vi "Test-Elevator Motors-Percent.vi"() -> ()   [LabVIEW 2014, in "Dev Elevator.lvlib"]
uses:
  Dev Robot/Dev Elevator/Dev Elevator.lvlib
  Robot Actor Framework/Trace/Trace Controller Class/Config.ctl
  Comp Motors with Encoders/Comp Motors with Encoders Class/Motor Controller Config.ctl
  Robot/Motor with Encoders/Motors with Encoders Class/Motors with Encoders Config.ctl
  Comp Motors with Encoders/Comp Motors with Encoders Class/Encoder Config.ctl
  Comp Trace Controller/Comp Trace Controller Class/Comp Trace Controller.lvclass
  Comp Pressure/Comp Pressure Class/Comp Pressure.lvclass
  <vilib>/Rock Robotics/WPI/Solenoid/WPI_SolenoidChannel.ctl
  Comp Motors with Encoders/Comp Motors with Encoders Class/Comp Motors with Encoders.lvclass
  <vilib>/Rock Robotics/WPI/DriverStation/WPI_DriverStationRobotMode2.ctl
  <vilib>/Rock Robotics/WPI/Solenoid/WPI_SolenoidValue.ctl
  Robot/Motor with Encoders/Motors with Encoders Messages/Set Rate (Percent) Msg/Set Rate (Percent) Msg.lvclass/Set Rate (Percent) Msg.ctl
  <vilib>/ActorFramework/Message Enqueuer/Message Enqueuer.lvclass/Message Enqueuer.ctl
  <vilib>/ActorFramework/Message Enqueuer/Enqueue.vi
  <vilib>/Rock Robotics/WPI/Solenoid/WPI_SolenoidOpenDouble.vi
  <vilib>/Rock Robotics/WPI/Solenoid/WPI_SolenoidSetEnum.vi
  <vilib>/ActorFramework/Message Priority Queue/Priority Enqueue.vi
  Robot/Motor with Encoders/Motors with Encoders Messages/Set Rate (Percent) Msg/Set Rate (Percent) Msg.lvclass
  <vilib>/ActorFramework/Stop Msg/Stop Msg.lvclass
  <vilib>/ActorFramework/Actor/Actor.lvclass
  Robot Actor Framework/Trace/Trace Controller Class/Trace Controller.lvclass
  Robot/Motor with Encoders/Motors with Encoders Class/Motors with Encoders.lvclass
panel:
  in  "Test Loop":u32=75
  in  "Encoder Config":T1={"P"=1.0, "D"=0.0, "F"=0.01, "I"=0.01, "Reverse Feedback Sensor"=FALSE, "Encoder Codes Per Rev"=256}
  out "Enable Tele":bool caption="Enabled Teleop"
  in  "Stop Test Loop 1":bool=TRUE
  in  "Finish Test":bool=TRUE
  in  "Start Test":bool=TRUE
  in  "Rate (Percent)":dbl(slide)=0.040816326530612165 scale=-1.0..1.0
  in  "Motos with Encoder Config":T2={"Counts  Per Revolution"=256, "Invert Encoder Direction"=FALSE, "Diameter of Revolution"=6.0, "Max RPM"=1500.0, "Encoder Control"=TRUE}
  in  "Slave Motor Controller Configs":T3[](array[typedef])
  in  "Master Motor Controller Config":T3={"Device Number"=7, "Invert Motor"=FALSE}
  in  "Trace Controller Config":T4={"Folder Pattern"="/media/sd%s1", "Starting Letter Position"=1, "Min Free Space (MB)"=50.0, "Max Folders to Check"=10, "Trace Level"=enum."Debug"} {"Min Free Space (MB)" format="%#_13g"}
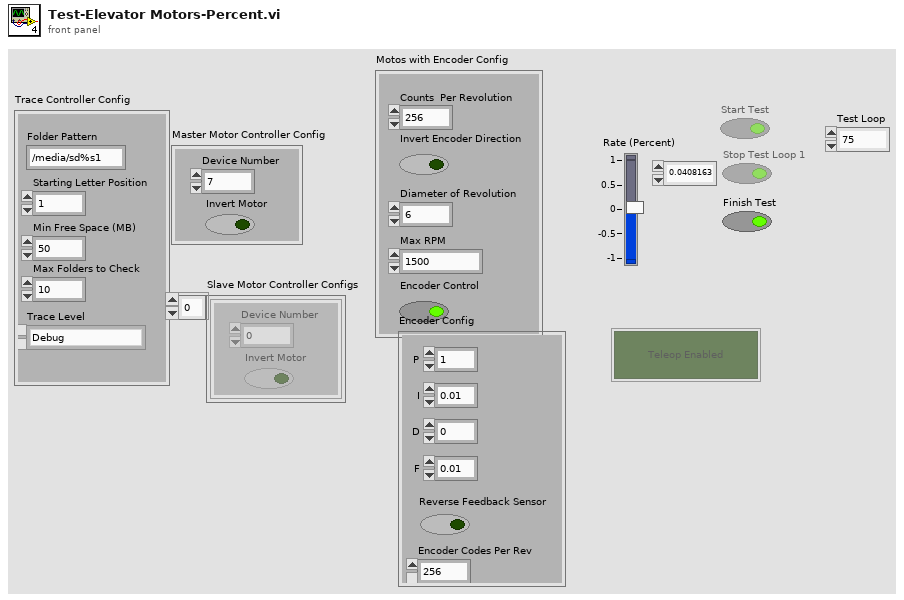
[diagram p1: front panel]
types:
  T1 = typedef "Comp Motors with Encoders.lvlib/Comp Motors with Encoders.lvclass/Encoder Config.ctl" = cluster{"P":dbl, "D":dbl, "F":dbl, "I":dbl, "Reverse Feedback Sensor":bool, "Encoder Codes Per Rev":u16}
  T2 = typedef "Motors with Encoders.lvlib/Motors with Encoders.lvclass/Motors with Encoders Config.ctl" = cluster{"Counts  Per Revolution":u32, "Invert Encoder Direction":bool, "Diameter of Revolution":dbl, "Max RPM":dbl, "Encoder Control":bool}
  T3 = typedef "Comp Motors with Encoders.lvlib/Comp Motors with Encoders.lvclass/Motor Controller Config.ctl" = cluster{"Device Number":u8, "Invert Motor":bool}
  T4 = typedef "Robot Actor Framework.lvlib/Trace.lvlib/Trace Controller.lvclass/Config.ctl" = cluster{"Folder Pattern":string, "Starting Letter Position":i32, "Min Free Space (MB)":dbl, "Max Folders to Check":u32, "Trace Level":enum16{"Critical", "Error", "Warning", "Informational", "Debug"}}
  T5 = typedef "WPI_SolenoidChannel.ctl" = enum8{"Solenoid 0", "Solenoid 1", "Solenoid 2", "Solenoid 3", "Solenoid 4", "Solenoid 5", "Solenoid 6", "Solenoid 7", "Invalid"}
  T6 = enum16{"Critical", "Error", "Warning", "Informational", "Debug"}
  T7 = enum8{"Enabled", "Disabled", "Disabled and Grayed Out"}
  T8 = typedef "WPI_DriverStationRobotMode2.ctl" = enum16{"Autonomous Disabled", "Autonomous Enabled", "Teleop Disabled", "Teleop Enabled", "Disconnected", "Finish", "Test Disabled", "Test Enabled", "Emergency Stopped"}
  T9 = typedef "WPI_SolenoidValue.ctl" = enum16{"Off", "On", "Forward", "Reverse"}
  T10 = typedef "WPI_SolenoidDevRef.ctl" = cluster{"DevStatus":errorcluster, "Pneumatics Control Module":u8, "Forward Solenoid Channel":T5, "Reverse Solenoid Channel":T5}
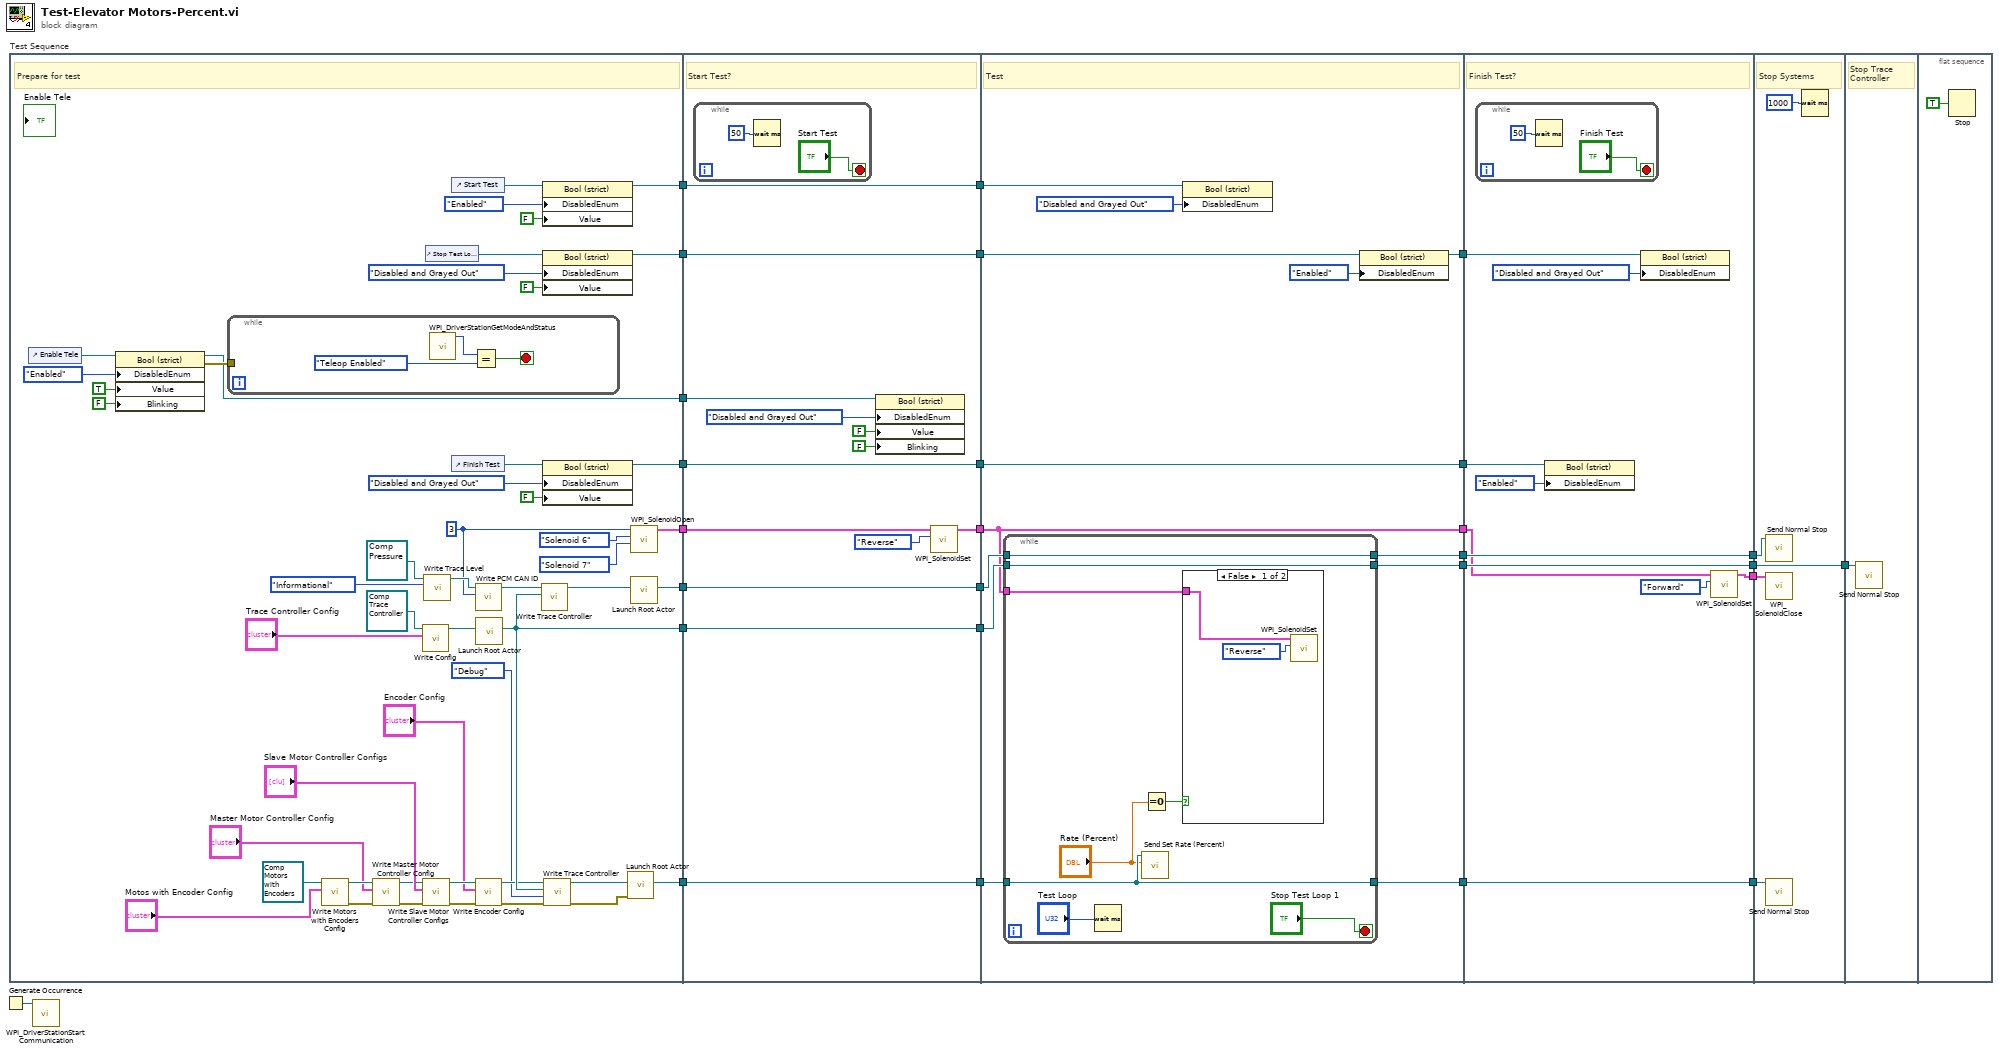
[diagram p0: block diagram]
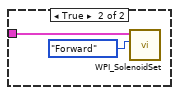
[diagram p2: hidden frame]
diagram:
  n1 = Generate Occurrence() -> (w27:refnum<k4>)
  n2 = flat-sequence "Test Sequence" {
    tunnel: [w59] -> w16
    tunnel: [w61] -> w15
    tunnel: [w60] -> w14
    tunnel: [w49] -> w13
    tunnel: [w48] -> w11
    tunnel: [w47] -> w6
    tunnel: [w41] -> w5
    tunnel: [w33] -> w4
    tunnel: [w92] -> w19
    tunnel: [w91] -> w18
    tunnel: [w90] -> w17
    tunnel: w16 -> [w92]
    tunnel: w15 -> [w91]
    tunnel: w14 -> [w90]
    tunnel: w13 -> [w89]
    tunnel: [w89] -> w12
    tunnel: w11 -> [w88]
    tunnel: [w88] -> w10
    tunnel: [w87] -> w7
    tunnel: w6 -> [w87]
    tunnel: w5 -> [w86]
    tunnel: w4 -> [w82]
    tunnel: [w81] -> w3
    tunnel: [w102] -> w22
    tunnel: [w104] -> w21
    tunnel: [w103] -> w20
    tunnel: w19 -> [w107]
    tunnel: w18 -> [w105]
    tunnel: w17 -> [w106]
    tunnel: w12 -> [w101]
    tunnel: w10 -> [w99]
    tunnel: [w97] -> w9
    tunnel: [w96] -> w8
    tunnel: w7 -> [w96]
    tunnel: w3 -> [w95]
    tunnel: [w95] -> w2
    tunnel: [w129] -> w25
    tunnel: [w128] -> w24
    tunnel: [w127] -> w23
    tunnel: w22 -> [w129]
    tunnel: w21 -> [w128]
    tunnel: w20 -> [w127]
    tunnel: w9 -> [w126]
    tunnel: w8 -> [w123]
    tunnel: w2 -> [w122]
    tunnel: [w121] -> w1
    tunnel: [w136] -> w26
    tunnel: w25 -> [w136]
    tunnel: w24 -> [w135]
    tunnel: w23 -> [w133]
    tunnel: w1 -> [w132]
    tunnel: w26 -> [w137]
    frame #0 {
      w34 = u8 3 ("PCM CAN ID")
      # "Prepare for test"
      n3 = control-ref of="Enable Tele"() -> (w46:refnum<vi>)
      n4 = property class="Bool (strict)"(reference=w46, "DisabledEnum"=T7."Enabled" ("Disabled"), "Value"=TRUE, "Blinking"=FALSE) -> (reference out=w41:refnum<vi>, error out=w43:errorcluster)  [unwired: 1 in]
      n5 = while {
        tunnel: w43 -> [_]
        stop <- w77 stop-if-true
        n6 = call <vilib>:"WPI_DriverStationGetModeAndStatus.vi"() -> ("Robot Mode"=w79:T8)  [unwired: 10 in, 1 out]
        n7 = Equal?(x=w79, y=WPI_DriverStationRobotMode2."Teleop Enabled") -> (x = y?=w77:bool)
      }
      n8 = call-dynamic "Write Motors with Encoders Config.vi"("Motors with Encoders Config"="Motos with Encoder Config", "Motors with Encoders in"=refnum<class "Comp Motors with Encoders.lvclass"> refnum ("Comp Motors with Encoders.lvlib:Comp Motors with Encoders.lvclass")) -> ("error out"=w68:errorcluster, "Motors with Encoders out"=w29:refnum<class "Comp Motors with Encoders.lvclass">)  [unwired: 8 in]
      n9 = call-dynamic "Write Master Motor Controller Config.vi"("error in (no error)"=w68, "Master Motor Controller Config"="Master Motor Controller Config", "Comp Motors with Encoders in"=w29) -> ("error out"=w69:errorcluster, "Comp Motors with Encoders out"=w65:refnum<class "Comp Motors with Encoders.lvclass">)  [unwired: 7 in]
      n10 = call-dynamic "Write Config.vi"("Config"="Trace Controller Config", "Trace Controller in"=refnum<class "Comp Trace Controller.lvclass"> refnum ("Comp Trace Controller.lvlib:Comp Trace Controller.lvclass")) -> ("Trace Controller out"=w64:refnum<class "Comp Trace Controller.lvclass">)  [unwired: 8 in, 1 out]
      n11 = call-dynamic "Write Slave Motor Controller Configs.vi"("error in (no error)"=w69, "Slave Motor Controller Configs"="Slave Motor Controller Configs", "Comp Motors with Encoders in"=w65) -> ("error out"=w38:errorcluster, "Comp Motors with Encoders out"=w40:refnum<class "Comp Motors with Encoders.lvclass">)  [unwired: 7 in]
      n12 = call-dynamic "Write Trace Level.vi"("Trace Level"=T6."Informational", "System Actor in"=refnum<class "Comp Pressure.lvclass"> refnum ("Comp Pressure.lvlib:Comp Pressure.lvclass")) -> ("System Actor out"=w74:refnum<class "Comp Pressure.lvclass">)  [unwired: 8 in, 1 out]
      n13 = control-ref of="Stop Test Loop 1"() -> (w53:refnum<vi>)
      n14 = control-ref of="Start Test"() -> (w58:refnum<vi>)
      n15 = control-ref of="Finish Test"() -> (w52:refnum<vi>)
      n16 = call-dynamic "Write PCM CAN ID.vi"("PCM CAN ID"=w34, "Comp Pressure in"=w74) -> ("Comp Pressure out"=w75:refnum<class "Comp Pressure.lvclass">)  [unwired: 8 in, 1 out]
      n17 = call-dynamic "Write Encoder Config.vi"("error in (no error)"=w38, "Encoder Config"="Encoder Config", "Comp Motors with Encoders in"=w40) -> ("error out"=w37:errorcluster, "Comp Motors with Encoders out"=w39:refnum<class "Comp Motors with Encoders.lvclass">)  [unwired: 7 in]
      n18 = call <vilib>:"Launch Root Actor.vi"("Actor"=w64) -> ("Actor's Enqueuer"=w60:refnum<class "Message Enqueuer.lvclass">)  [unwired: 9 in, 1 out]
      n19 = call-dynamic "Write Trace Controller.vi"("Trace Controller"=w60, "System Actor in"=w75) -> ("System Actor out"=w76:refnum<class "Comp Pressure.lvclass">)  [unwired: 8 in, 1 out]
      n20 = property class="Bool (strict)"(reference=w58, "DisabledEnum"=T7."Enabled" ("Disabled"), "Value"=FALSE) -> (reference out=w49:refnum<vi>)  [unwired: 1 in, 1 out]
      n21 = property class="Bool (strict)"(reference=w53, "DisabledEnum"=T7."Disabled and Grayed Out" ("Disabled"), "Value"=FALSE) -> (reference out=w48:refnum<vi>)  [unwired: 1 in, 1 out]
      n22 = property class="Bool (strict)"(reference=w52, "DisabledEnum"=T7."Disabled and Grayed Out" ("Disabled"), "Value"=FALSE) -> (reference out=w47:refnum<vi>)  [unwired: 1 in, 1 out]
      n23 = call-dynamic "Write Trace Controller.vi"("error in (no error)"=w37, "Trace Level"=T6."Debug", "Trace Controller"=w60, "System Actor in"=w39) -> ("error out"=w71:errorcluster, "System Actor out"=w70:refnum<class "Comp Motors with Encoders.lvclass">)  [unwired: 6 in]
      n24 = call <vilib>:"Launch Root Actor.vi"("error in (no error)"=w71, "Actor"=w70) -> ("Actor's Enqueuer"=w59:refnum<class "Message Enqueuer.lvclass">)  [unwired: 8 in, 1 out]
      n25 = call-poly <vilib>:"WPI_SolenoidOpen.vi"("Reverse Solenoid Channel"=WPI_SolenoidChannel."Solenoid 7", "Forward Solenoid Channel"=WPI_SolenoidChannel."Solenoid 6", "Pneumatics Control Module (0)"=w34) -> ("SolenoidDevRef"=w33:T10)  [unwired: 7 in, 1 out]
      n26 = call <vilib>:"Launch Root Actor.vi"("Actor"=w76) -> ("Actor's Enqueuer"=w61:refnum<class "Message Enqueuer.lvclass">)  [unwired: 9 in, 1 out]
    }
    frame #1 {
      # "Start Test?"
      n27 = while {
        stop <- "Start Test" stop-if-true
        n28 = Wait (ms)(milliseconds to wait=u32 50) -> ()  [unwired: 1 out]
      }
      n29 = property class="Bool (strict)"(reference=w86, "DisabledEnum"=T7."Disabled and Grayed Out" ("Disabled"), "Value"=FALSE, "Blinking"=FALSE) -> ()  [unwired: 1 in, 2 out]
      n30 = call-poly <vilib>:"WPI_SolenoidSet.vi"("Value"=WPI_SolenoidValue."Reverse", "SolenoidDevRef"=w82) -> ("SolenoidDevRef"=w81:T10)  [unwired: 8 in, 1 out]
    }
    frame #2 {
      # "Test"
      n31 = while {
        tunnel: w106 -> [w114]
        tunnel: [w114] -> w102
        tunnel: w107 -> [w111]
        tunnel: [w111] -> w104
        tunnel: w105 -> [w113]
        tunnel: [w113] -> w103
        tunnel: w95 -> [w110]
        stop <- "Stop Test Loop 1" stop-if-true
        n32 = Wait (ms)(milliseconds to wait="Test Loop") -> ()  [unwired: 1 out]
        n33 = call "Send Set Rate (Percent).vi"("Rate (Percentage)"="Rate (Percent)", "Message Enqueuer"=w111) -> ()  [unwired: 8 in, 2 out]
        n34 = Equal To 0?(x="Rate (Percent)") -> (x = 0?=w108:bool)
        n35 = case shown="False" w108 {
          tunnel: w110 -> [w117 w119]
          frame False {
            n36 = call-poly <vilib>:"WPI_SolenoidSet.vi"("Value"=WPI_SolenoidValue."Reverse", "SolenoidDevRef"=w117) -> ()  [unwired: 8 in, 2 out]
          }
          frame True {
            n37 = call-poly <vilib>:"WPI_SolenoidSet.vi"("Value"=WPI_SolenoidValue."Forward", "SolenoidDevRef"=w119) -> ()  [unwired: 8 in, 2 out]
          }
        }
      }
      n38 = property class="Bool (strict)"(reference=w101, "DisabledEnum"=T7."Disabled and Grayed Out" ("Disabled")) -> ()  [unwired: 1 in, 2 out]
      n39 = property class="Bool (strict)"(reference=w99, "DisabledEnum"=T7."Enabled" ("Disabled")) -> (reference out=w97:refnum<vi>)  [unwired: 1 in, 1 out]
    }
    frame #3 {
      # "Finish Test?"
      n40 = while {
        stop <- "Finish Test" stop-if-true
        n41 = Wait (ms)(milliseconds to wait=u32 50) -> ()  [unwired: 1 out]
      }
      n42 = property class="Bool (strict)"(reference=w123, "DisabledEnum"=T7."Enabled" ("Disabled")) -> ()  [unwired: 1 in, 2 out]
      n43 = property class="Bool (strict)"(reference=w126, "DisabledEnum"=T7."Disabled and Grayed Out" ("Disabled")) -> ()  [unwired: 1 in, 2 out]
      n44 = call-poly <vilib>:"WPI_SolenoidSet.vi"("Value"=WPI_SolenoidValue."Forward", "SolenoidDevRef"=w122) -> ("SolenoidDevRef"=w121:T10)  [unwired: 8 in, 1 out]
    }
    frame #4 {
      # "Stop Systems"
      n45 = call <vilib>:"Send Normal Stop.vi"("Message Enqueuer"=w133) -> ()  [unwired: 10 in, 1 out]
      n46 = call <vilib>:"WPI_SolenoidClose.vi"("SolenoidDevRef"=w132) -> ()  [unwired: 10 in, 1 out]
      n47 = call <vilib>:"Send Normal Stop.vi"("Message Enqueuer"=w135) -> ()  [unwired: 10 in, 1 out]
      n48 = Wait (ms)(milliseconds to wait=u32 1000) -> ()  [unwired: 1 out]
    }
    frame #5 {
      # "Stop Trace Controller"
      n49 = call <vilib>:"Send Normal Stop.vi"("Message Enqueuer"=w137) -> ()  [unwired: 10 in, 1 out]
    }
    frame #6 {
      n50 = Stop(stop? (T)=TRUE) -> ()
    }
  }
  n51 = call <vilib>:"WPI_DriverStationStart Communication.vi"("occurrence"=w27) -> ()  [unwired: 1 in, 10 out]
